vi "arb_transmit.vi"(8 "error in (no error)":errorcluster, 10 "Waveform Graph":waveform(dbl)[](graph)=[{"t0"=timestamp(0 s since 1904-01-01), "dt"=0.01, "Y"=array[1000 elements]}, {"t0"=timestamp(0 s since 1904-01-01), "dt"=0.01, "Y"=array[1000 elements]}, {"t0"=timestamp(0 s since 1904-01-01), "dt"=0.01, "Y"=array[1000 elements]}, {"t0"=timestamp(0 s since 1904-01-01), "dt"=0.01, "Y"=array[1000 elements]}], 11 "output":T1[](array[typedef]) {"channel" items=["1", "2"]}) -> (0 "error out":errorcluster)   [LabVIEW 2017, in "wf.lvlib"]
uses:
  wf.lvlib
  wf_channel.ctl
  <vilib>/Instr/_visa.llb/Select Event Type.ctl
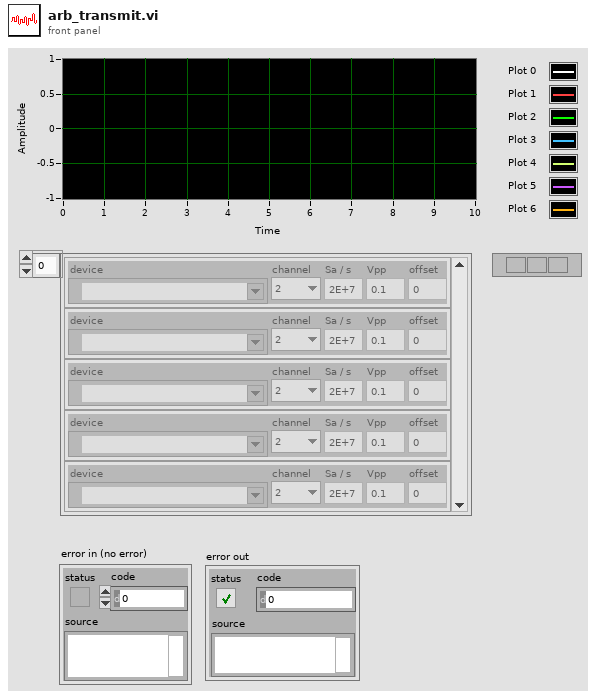
[diagram p1: front panel]
types:
  T1 = typedef "wf.lvlib/wf_channel.ctl" = cluster{"device":refnum<visa-resource-name>, "channel":u8, "Sa / s":dbl, "Vpp":dbl, "offset":dbl}
  T2 = typedef "Select Event Type.ctl" = u32
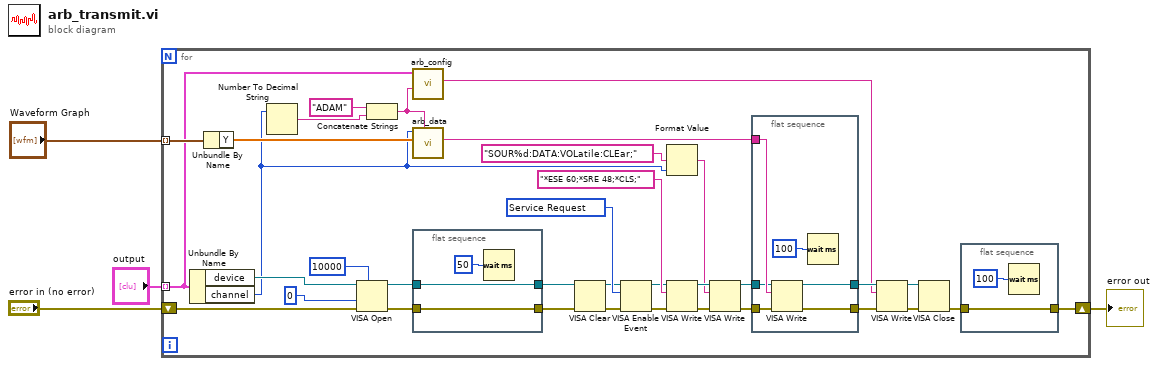
[diagram p0: block diagram]
diagram:
  n1 = for {
    tunnel: "Waveform Graph" -> [w39] mode=indexing
    tunnel: "output" -> [w6] mode=indexing
    shift-right: [w16] -> w3
    shift-left: "error in (no error)" -> [w32]
    w22 = T2 1073684491 items=["Service Request"=1073684491, "Trigger"=3221168138, "Clear"=1073684493, "VXI Signal"=1073684512, "VXI/VME Interrupt"=3221168161, "VXI/VME Sysfail"=1073684509, "VXI/VME Sysreset"=1073684510, "GPIB CIC"=1073684498, "GPIB Talk"=1073684499, "GPIB Listen"=1073684500, "PXI Interrupt"=1073684514, "Serial Break"=1073684515, "Serial TermChar"=1073684516, "Serial CTS"=1073684521, "Serial DSR"=1073684522, "Serial DCD"=1073684524, "Serial RI"=1073684526, "Serial Character"=1073684533, "USB Interrupt"=1073684535, "All Enabled"=1073709055] ("Event Type")
    n2 = Unbundle By Name(w6) -> ("device"=w33:refnum<visa-resource-name>, "channel"=w5:u8)
    n3 = Unbundle By Name(w39) -> ("Y"=w31:dbl[])
    n4 = Number To Decimal String(number=w5) -> (decimal integer string=w29:string)  [unwired: 1 in]
    n5 = VISA Open(timeout (0)=u32 10000 ("VISA Open timeout (0)"), access mode=u32 0, error in (no error)=w32, VISA resource name=w33) -> (VISA resource name=w25:refnum<visa-resource-name>, error out=w24:errorcluster)  [unwired: 1 out]
    n6 = Concatenate Strings("ADAM", w29) -> (w8:string)
    n7 = call "arb_config.vi"("name"=w8, "wf"=w6) -> ("cmd"=w7:string)  [unwired: 8 in, 1 out]
    n8 = call "arb_data.vi"("name"=w8, "wf"=w31, "channel"=w5) -> ("cmd"=w30:string)  [unwired: 8 in]
    n9 = flat-sequence {
      tunnel: [w49] -> w18
      tunnel: w25 -> [w49]
      tunnel: [w48] -> w19
      tunnel: w24 -> [w48]
      frame #0 {
        n10 = Wait (ms)(milliseconds to wait=u32 50) -> ()  [unwired: 1 out]
      }
    }
    n11 = VISA Clear(VISA resource name=w18, error in (no error)=w19) -> (VISA resource name out=w21:refnum<visa-resource-name>, error out=w20:errorcluster)
    n12 = VISA Enable Event(8:w20, 10:w22, 11:w21) -> (0:w12:errorcluster, 3:w14:refnum<visa-resource-name>)  [unwired: 1 in]
    n13 = Format Value(format string="SOUR%d:DATA:VOLatile:CLEar;", value (0)=w5) -> (output string=w9:string)  [unwired: 1 in]
    n14 = VISA Write(VISA resource name=w14, write buffer="*ESE 60;*SRE 48;*CLS;" ("Default Setup String"), error in (no error)=w12) -> (VISA resource name out=w13:refnum<visa-resource-name>, error out=w11:errorcluster)  [unwired: 1 out]
    n15 = VISA Write(VISA resource name=w13, write buffer=w9, error in (no error)=w11) -> (VISA resource name out=w26:refnum<visa-resource-name>, error out=w27:errorcluster)  [unwired: 1 out]
    n16 = flat-sequence {
      tunnel: [w45] -> w36
      tunnel: [w44] -> w35
      tunnel: w30 -> [w43]
      tunnel: w27 -> [w42]
      tunnel: w26 -> [w41]
      frame #0 {
        n17 = VISA Write(VISA resource name=w41, write buffer=w43, error in (no error)=w42) -> (VISA resource name out=w44:refnum<visa-resource-name>, error out=w45:errorcluster)  [unwired: 1 out]
        n18 = Wait (ms)(milliseconds to wait=u32 100) -> ()  [unwired: 1 out]
      }
    }
    n19 = VISA Write(VISA resource name=w35, write buffer=w7, error in (no error)=w36) -> (VISA resource name out=w38:refnum<visa-resource-name>, error out=w37:errorcluster)  [unwired: 1 out]
    n20 = VISA Close(VISA resource name=w38, error in (no error)=w37) -> (error out=w17:errorcluster)
    n21 = flat-sequence {
      tunnel: [w46] -> w16
      tunnel: w17 -> [w46]
      frame #0 {
        n22 = Wait (ms)(milliseconds to wait=u32 100) -> ()  [unwired: 1 out]
      }
    }
  }
  "error out" <- w3
